vi "gen j disorder.vi"(7 "Input":T1={"Step width"=0.2, "App"=0.1, "Array"=[1.0078411649904462, 1.0078411649904462, 0.9846991573254764, 0.9846991573254764, 0.9978814600222632, 0.9978814600222632, 0.9723089162683902, 0.9723089162683902, 1.011631648566163, 1.011631648566163]}, 9 "Step width":dbl=0.2, 10 "App":dbl=0.1, 11 "Points":i32=10) -> (3 "Output":T1={"Step width"=0.2, "App"=0.1, "Array"=[1.0078411649904462, 1.0078411649904462, 0.9846991573254764, 0.9846991573254764, 0.9978814600222632, 0.9978814600222632, 0.9723089162683902, 0.9723089162683902, 1.011631648566163, 1.011631648566163]})   [LabVIEW 2023]
panel:
  in  "Set":bool
  in  "Generate":bool
  out "Disorder Pattern":dbl[](graph)=[1.0078411649904462, 1.0078411649904462, 0.9846991573254764, 0.9846991573254764, 0.9978814600222632, 0.9978814600222632, 0.9723089162683902, 0.9723089162683902, 1.011631648566163, 1.011631648566163]
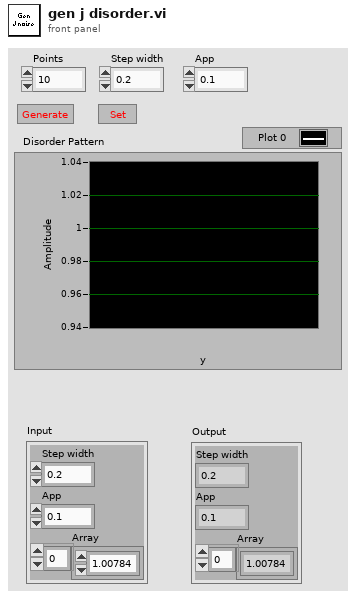
[diagram p1: front panel]
types:
  T1 = cluster{"Step width":dbl, "App":dbl, "Array":dbl[]}
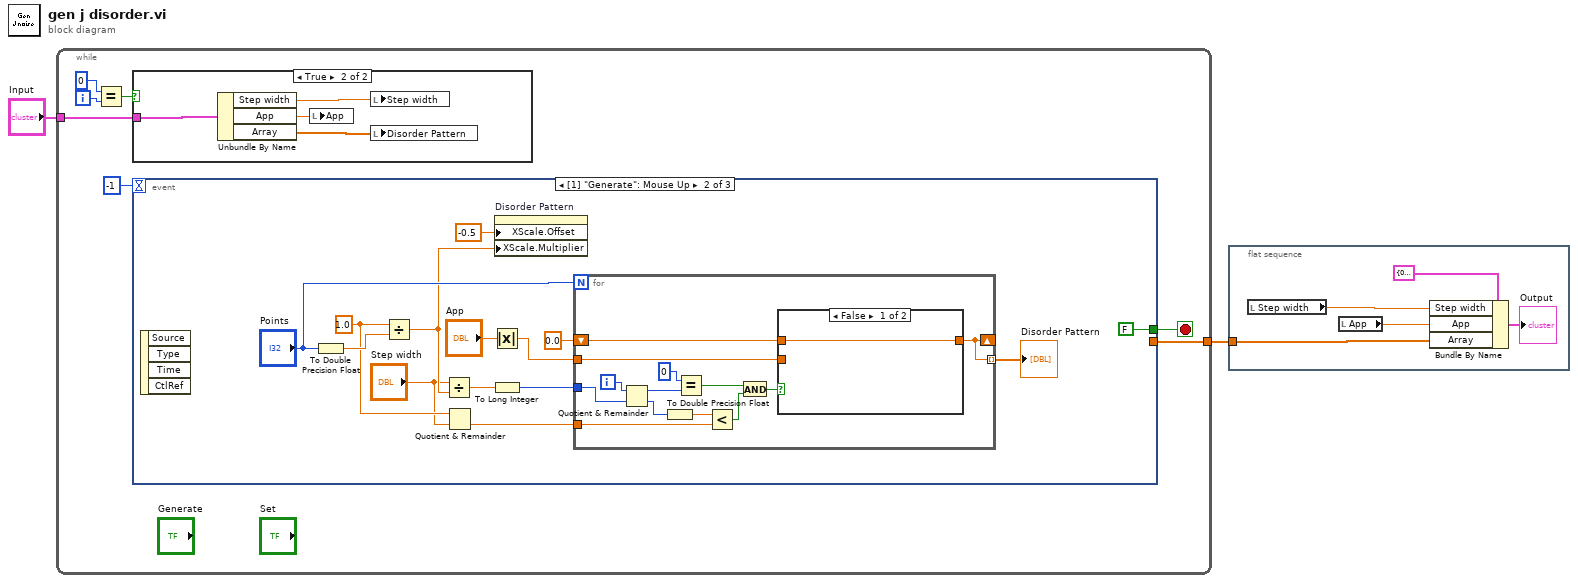
[diagram p0: block diagram]
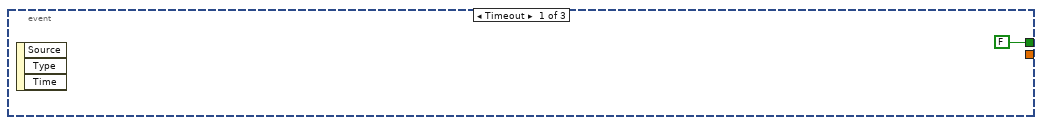
[diagram p3: hidden frame]
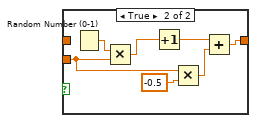
[diagram p4: hidden frame]
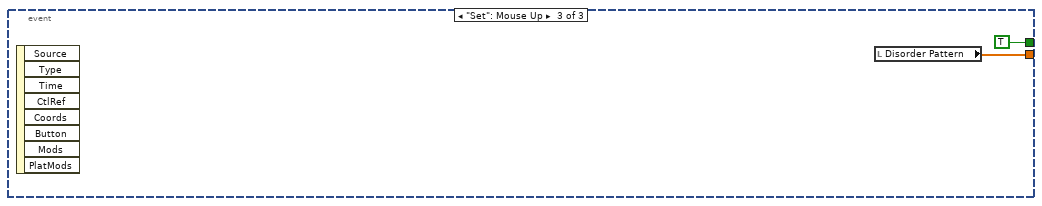
[diagram p5: hidden frame]
diagram:
  n1 = while {
    tunnel: [w7] -> w2
    tunnel: "Input" -> [w3]
    i -> [w6]
    stop <- w8 stop-if-true
    n2 = Equal?(x=0, y=w6) -> (x = y?=w4:bool)
    n3 = case shown="True" w4 {
      tunnel: w3 -> [_ w13]
      frame False {
      }
      frame True {
        n4 = Unbundle By Name(w13) -> ("Step width"=w12:dbl, "App"=w11:dbl, "Array"=w10:dbl[])
        n5 = local write "App"(w11) -> ()
        n6 = local write "Step width"(w12) -> ()
        n7 = local write "Disorder Pattern"(w10) -> ()
      }
    }
    n8 = event shown="[1] \"Generate\": Mouse Up" {
      selector: _ -> [_ _ _]
      dyn-events: _ -> [_ _ _]
      timeout: -1 -> [_ _ _]
      tunnel: [FALSE FALSE TRUE] -> w8
      tunnel: [_ _ w51] -> w7
      event Timeout {
        n9 = event-data() -> ()  [unwired: 1 in, 3 out]
      }
      event "Generate": Mouse Up {
        w17 = 1.0 ("x")
        n10 = event-data() -> ()  [unwired: 1 in, 4 out]
        n11 = To Double Precision Float(number="Points") -> (double precision float=w23:dbl)
        n12 = Divide(x=w17, y=w23) -> (x/y=w18:dbl)
        n13 = Divide(x="Step width", y=w18) -> (x/y=w24:dbl)
        n14 = Quotient & Remainder(x=w17, y="Step width") -> (floor(x/y)=w15:dbl)  [unwired: 1 out]
        n15 = Absolute Value(x="App") -> (abs(x)=w28:dbl)
        n16 = To Long Integer(number=w24) -> (32bit integer=w26:i32)
        n17 = property on="Disorder Pattern" class="WFGraph (strict)"("XScale.Offset"=-0.5, "XScale.Multiplier"=w18) -> ()  [unwired: 2 in, 2 out]
        n18 = for {
          N: "Points" -> [_]
          tunnel: w26 -> [w41]
          tunnel: w28 -> [w39]
          shift-right: [w37] -> _
          shift-left: 0.0 -> [w38]
          tunnel: [w37] -> w21 mode=indexing
          tunnel: w15 -> [w33]
          i -> [w34]
          n19 = Quotient & Remainder(x=w34, y=w41) -> (x-y*floor(x/y)=w36:i32, floor(x/y)=w29:i32)
          n20 = To Double Precision Float(number=w29) -> (double precision float=w32:dbl)
          n21 = Equal?(x=0, y=w36) -> (x = y?=w35:bool)
          n22 = Less?(x=w32, y=w33) -> (x < y?=w31:bool)
          n23 = And(x=w35, y=w31) -> (x .and. y?=w30:bool)
          n24 = case shown="False" w30 {
            tunnel: w39 -> [_ w47]
            tunnel: [w42 w43] -> w37
            tunnel: w38 -> [w42 _]
            frame False {
            }
            frame True {
              n25 = Random Number (0-1)() -> (number: 0 to 1=w49:dbl)
              n26 = Multiply(x=w49, y=w47) -> (x*y=w48:dbl)
              n27 = Increment(x=w48) -> (x+1=w45:dbl)
              n28 = Multiply(x=w47, y=-0.5) -> (x*y=w44:dbl)
              n29 = Add(x=w45, y=w44) -> (x+y=w43:dbl)
            }
          }
        }
        "Disorder Pattern" <- w21
      }
      event "Set": Mouse Up {
        n30 = event-data() -> ()  [unwired: 1 in, 8 out]
        n31 = local read "Disorder Pattern"() -> (w51:dbl[])
      }
    }
  }
  n32 = flat-sequence {
    tunnel: w2 -> [w54]
    frame #0 {
      n33 = local read "Step width"() -> (w53:dbl)
      n34 = local read "App"() -> (w52:dbl)
      n35 = Bundle By Name(cluster=T1 {"Step width"=0.2, "App"=0.1, "Array"=[1.0078411649904462, 1.0078411649904462, 0.9846991573254764, 0.9846991573254764, 0.9978814600222632, 0.9978814600222632, 0.9723089162683902, 0.9723089162683902, 1.011631648566163, 1.011631648566163]} ("Cluster 2"), "Step width"=w53, "App"=w52, "Array"=w54) -> (→"Output":T1)
    }
  }
